vi "Set_Configuration_Keithley.vi"(0 "Filename (.ini)":string="Config_Ver_1\\Keithley_params.ini", 1 "Arm Layer Params In":T12={"Bypass Arm Layer\nInput Trigger?"=FALSE, "Input Trig Source"=enum."Trigger Link", "Input Trig Link Line"=enum."1", "Arm Timer Interval (s)"=0.001, "Output Trig Mode"=enum."No Trig Out", "Output Trig Link Line"=enum."1"} {"Arm Timer Interval (s)" min=0.001 max=99999.999 step=0.001 format="%.3f"}, 2 "List Sweep Params In":T2={"Abort On\nCompliance?"=FALSE, "List Sweep Steps"=[{"Current Level (A)"=0.0, "Source Delay (s)"=0.001, "Voltage Limit (V)"=100.0}, {"Current Level (A)"=0.1, "Source Delay (s)"=1.0, "Voltage Limit (V)"=100.0}]} {"List Sweep Steps"."Current Level (A)" min=-0.105 max=0.105 format="%.4p"; "List Sweep Steps"."Source Delay (s)" min=0.001 max=1000.0 step=0.001 format="%.3f"; "List Sweep Steps"."Voltage Limit (V)" min=0.1 max=105.0 step=0.01 format="%.2p"}, 3 "error in":errorcluster, 4 "Display Params":T1, 5 "Trig Layer Params In":T8={"Input Trig Source"=enum."Trigger Link", "Input Trig Link Line"=enum."1", "Output Trig Mode"=enum."Source Turn On", "Output Trig Link Line"=enum."2"}) -> (10 "error out":errorcluster)   [LabVIEW 2021]
uses:
  <instrlib>/Keithley 622x LV 2009/Configure/Trigger/Typedefs/KE622x -- Arm Layer Params.ctl
  <instrlib>/Keithley 622x LV 2009/Configure/Trigger/Low Level/Typedefs/KE622x -- Arm Source.ctl
  <instrlib>/Keithley 622x LV 2009/Configure/Trigger/Low Level/Typedefs/KE622x -- Trig Link Line.ctl
  <instrlib>/Keithley 622x LV 2009/Configure/Trigger/Low Level/Typedefs/KE622x -- Arm Timer Interval.ctl
  <instrlib>/Keithley 622x LV 2009/Configure/Trigger/Low Level/Typedefs/KE622x -- Arm Output Mode.ctl
  <instrlib>/Keithley 622x LV 2009/Configure/Trigger/Typedefs/KE622x -- Trig Layer Params.ctl
  <instrlib>/Keithley 622x LV 2009/Configure/Trigger/Low Level/Typedefs/KE622x -- Trig Source.ctl
  <instrlib>/Keithley 622x LV 2009/Configure/Trigger/Low Level/Typedefs/KE622x -- Trig Output Mode.ctl
  <instrlib>/Keithley 622x LV 2009/Configure/Source/Typedefs/KE622x -- List Sweep Params.ctl
  <instrlib>/Keithley 622x LV 2009/Configure/Source/Typedefs/KE622x -- List Sweep Steps.ctl
  <instrlib>/Keithley 622x LV 2009/Configure/Source/Typedefs/KE622x -- List Sweep Step.ctl
  <instrlib>/Keithley 622x LV 2009/Configure/Source/Typedefs/KE622x -- Current Level.ctl
  <instrlib>/Keithley 622x LV 2009/Configure/Source/Typedefs/KE622x -- Source Delay.ctl
  <instrlib>/Keithley 622x LV 2009/Configure/Source/Typedefs/KE622x -- Voltage Limit.ctl
  <instrlib>/Keithley 622x LV 2009/Configure/Display/Typedefs/KE622x -- Display Params.ctl
  <vilib>/Utility/config.llb/NI_LVConfig.lvlib
  <instrlib>/Keithley 622x LV 2009/Keithley 622x.lvlib
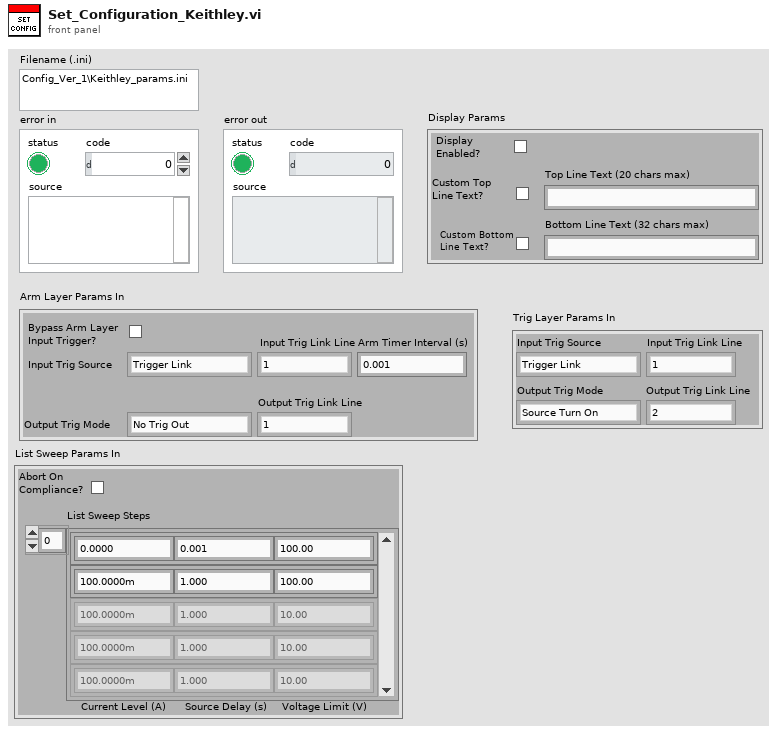
[diagram p1: front panel]
types:
  T1 = typedef "Keithley 622x.lvlib/KE622x -- Display Params.ctl" = cluster{"Display\nEnabled?":bool, "Custom Top\nLine Text?":bool, "Top Line Text (20 chars max)":string, "Custom Bottom\nLine Text?":bool, "Bottom Line Text (32 chars max)":string}
  T2 = typedef "Keithley 622x.lvlib/KE622x -- List Sweep Params.ctl" = cluster{"Abort On\nCompliance?":bool, "List Sweep Steps":T3}
  T3 = typedef "Keithley 622x.lvlib/KE622x -- List Sweep Steps.ctl" = T4[]
  T4 = typedef "Keithley 622x.lvlib/KE622x -- List Sweep Step.ctl" = cluster{"Current Level (A)":T5, "Source Delay (s)":T6, "Voltage Limit (V)":T7}
  T5 = typedef "Keithley 622x.lvlib/KE622x -- Current Level.ctl" = dbl
  T6 = typedef "Keithley 622x.lvlib/KE622x -- Source Delay.ctl" = dbl
  T7 = typedef "Keithley 622x.lvlib/KE622x -- Voltage Limit.ctl" = dbl
  T8 = typedef "Keithley 622x.lvlib/KE622x -- Trig Layer Params.ctl" = cluster{"Input Trig Source":T9, "Input Trig Link Line":T10, "Output Trig Mode":T11, "Output Trig Link Line":T10}
  T9 = typedef "Keithley 622x.lvlib/KE622x -- Trig Source.ctl" = enum16{"Immediate", "Trigger Link"}
  T10 = typedef "Keithley 622x.lvlib/KE622x -- Trig Link Line.ctl" = enum16{"1", "2", "3", "4", "5", "6"}
  T11 = typedef "Keithley 622x.lvlib/KE622x -- Trig Output Mode.ctl" = enum16{"No Trig Out", "Source Turn On", "After Source Delay"}
  T12 = typedef "Keithley 622x.lvlib/KE622x -- Arm Layer Params.ctl" = cluster{"Bypass Arm Layer\nInput Trigger?":bool, "Input Trig Source":T13, "Input Trig Link Line":T10, "Arm Timer Interval (s)":T14, "Output Trig Mode":T15, "Output Trig Link Line":T10}
  T13 = typedef "Keithley 622x.lvlib/KE622x -- Arm Source.ctl" = enum16{"Immediate", "Bus (*TRG)", "Timer", "Manual", "Trigger Link", "SOT Falling Edge", "SOT Rising Edge", "SOT Either Edge"}
  T14 = typedef "Keithley 622x.lvlib/KE622x -- Arm Timer Interval.ctl" = dbl
  T15 = typedef "Keithley 622x.lvlib/KE622x -- Arm Output Mode.ctl" = enum16{"No Trig Out", "Trig Out On Enter Arm", "Trig Out On Exit Arm"}
  T16 = typedef "NI_LVConfig.lvlib/Config Data RefNum.ctl" = refnum<k1>
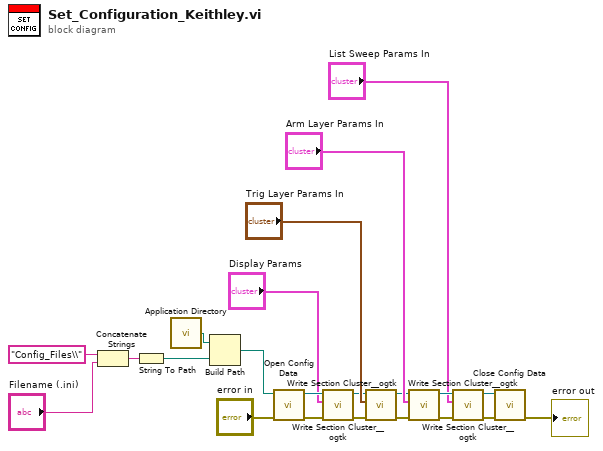
[diagram p0: block diagram]
diagram:
  n1 = Concatenate Strings("Config_Files\\" ("string"), "Filename (.ini)") -> (w17:string)
  n2 = String To Path(string=w17) -> (path=w20:path)
  n3 = call <vilib>:"Application Directory.vi"() -> ("Application Directory"=w22:path)
  n4 = Build Path(base path=w22, name or relative path=w20) -> (appended path=w21:path)
  n5 = call <vilib>:"Open Config Data.vi"("error in (no error)"="error in", "configuration file path"=w21) -> ("error out"=w5:errorcluster, "refnum"=w6:T16)  [unwired: 7 in, 1 out]
  n6 = call <userlib>:"Write Section Cluster__ogtk.vi"("error in (no error)"=w5, "Section Formatted Cluster"="Display Params", "refnum"=w6) -> ("error out"=w3:errorcluster, "dup refnum"=w4:T16)  [unwired: 7 in]
  n7 = call <userlib>:"Write Section Cluster__ogtk.vi"("error in (no error)"=w3, "Section Formatted Cluster"="Trig Layer Params In", "refnum"=w4) -> ("error out"=w14:errorcluster, "dup refnum"=w15:T16)  [unwired: 7 in]
  n8 = call <userlib>:"Write Section Cluster__ogtk.vi"("error in (no error)"=w14, "Section Formatted Cluster"="Arm Layer Params In", "refnum"=w15) -> ("error out"=w10:errorcluster, "dup refnum"=w11:T16)  [unwired: 7 in]
  n9 = call <userlib>:"Write Section Cluster__ogtk.vi"("error in (no error)"=w10, "Section Formatted Cluster"="List Sweep Params In", "refnum"=w11) -> ("error out"=w9:errorcluster, "dup refnum"=w8:T16)  [unwired: 7 in]
  n10 = call <vilib>:"Close Config Data.vi"("error in (no error)"=w9, "refnum"=w8) -> ("error out"=→"error out":errorcluster)  [unwired: 8 in, 1 out]
